vi "Get Error.vi"(11 "Template Queue in":refnum<class "Template Queue.lvclass">) -> (2 "Error":errorcluster)   [LabVIEW 2021, in "Template Queue.lvlib" / "Template Queue.lvclass"]
uses:
  Template Queue.lvclass
  Template Queue.lvclass/Template Queue.ctl
  <vilib>/Nathan Davis/jettl/jettl/Queue/Queue.lvclass
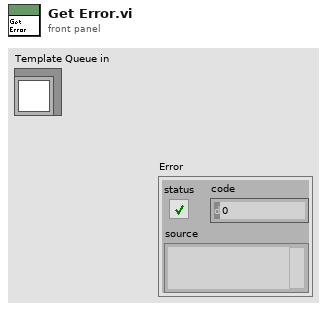
[diagram p1: front panel]
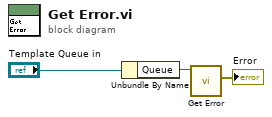
[diagram p0: block diagram]
diagram:
  n1 = Unbundle By Name("Template Queue in") -> ("Queue"=w2:refnum<class "Queue.lvclass">)
  n2 = call-dynamic "Get Error.vi"("jettl in"=w2) -> ("Error"=→"Error":errorcluster)  [unwired: 10 in]
